vi "GOMDBTS2048 integral Get Saturation.vi"(8 "error in (no error)":errorcluster, 11 "handle":i32) -> (0 "error out":errorcluster, 1 "function return":i32, 2 "saturation15bit":dbl, 3 "saturationPercent":dbl)   [LabVIEW 2015, in "GOMDBTS2048.lvlib"]
doc: "GOBTS2048DLL int __stdcall GOMDBTS2048_integralGetSaturation(int handle, double* saturationPercent, double* saturation15bit);"
uses:
  GOMDBTS2048.lvlib
  runtime/GOMDBTS2048.dll
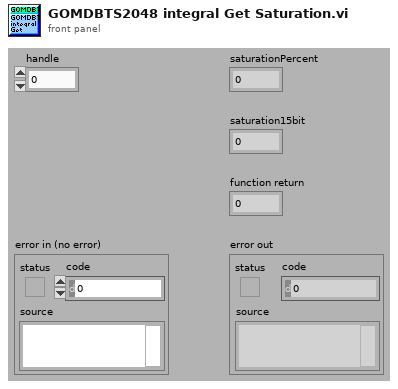
[diagram p1: front panel]
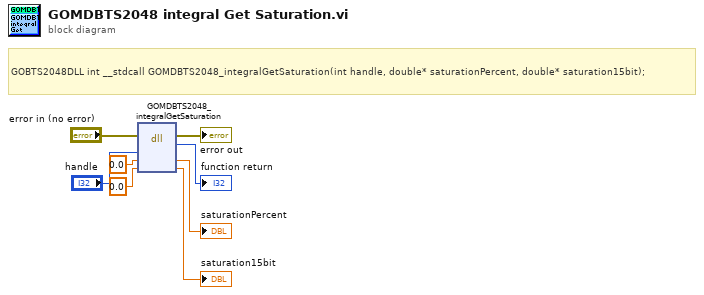
[diagram p0: block diagram]
diagram:
  # "GOBTS2048DLL int __stdcall GOMDBTS2048_integralGetSaturation(int handle, double* saturationPercent, double* saturation15bit);"
  n1 = dll-call lib="C:/Users/rkoch/Documents/GO_Library/runtime/GOMDBTS2048.*" fn="GOMDBTS2048_integralGetSaturation"(error in="error in (no error)", "handle"="handle", "saturationPercent"=0.0, "saturation15bit"=0.0) -> (error out=→"error out":errorcluster, →"function return":i32, "saturationPercent"=→"saturationPercent":dbl, "saturation15bit"=→"saturation15bit":dbl)  [unwired: 3 in, 1 out]
